vi "Facade 1.vi"(0 "Data In":T7, 2 "Display State In":T4, 3 "Container State":T6) -> (6 "Data Out":T7, 7 "Display State Out":T4, 8 "Action":T3)   [LabVIEW 2012, in "paint Xcontrol.xctl"]
doc: "This VI defines the appearance and behavior of the Paint XControl. The front panel of the Facade VI defines the appearance of the XControl. The block diagram of the Facade VI describes the behavior of the XControl, using an Event Structure to defined respones to various events that can occur on the XControl."
uses:
  paint Xcontrol.xctl
  Data 1.ctl
  <vilib>/_xctls/Container State.ctl
  State 1.ctl
  controls/tool enum.ctl
  <vilib>/_xctls/Action.ctl
  <vilib>/Utility/cursorutil.llb/Set Cursor (Icon Pict).vi
  Instance           4 16Saved   Facade 1 .vi
  <vilib>/_xctls/XControlSupport.lvlib
panel:
  in  "Fill Shapes":bool
  in  "Line Style":T1={"Width"=1, "Style"=enum."Solid"}
  in  "Text String":string
  in  "Tool":T2(radio)
  in  "Color":u32(colorbox)
  out "Picture":picture
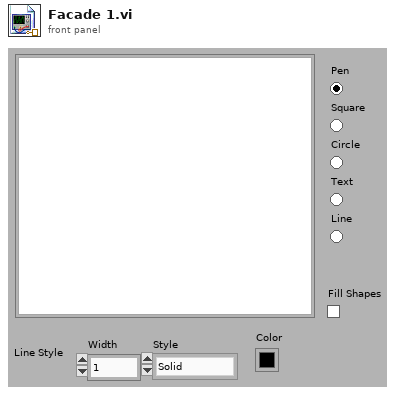
[diagram p1: front panel]
types:
  T1 = cluster{"Width":u16, "Style":enum32{"Solid", "Dash", "Dot", "DashDot", "DashDotDot"}}
  T2 = enum32{"Pen", "Square", "Circle", "Text", "Line"}
  T3 = typedef "XControlSupport.lvlib/Action.ctl" = cluster{"Data Changed?":bool, "State Changed?":bool, "Action Name":string}
  T4 = typedef "paint Xcontrol.xctl/State 1.ctl" = cluster{"Mouse Down?":bool, "Tool":T5, "Start Coords":cluster{"Horizontal":i32, "Vertical":i32}}
  T5 = typedef "paint Xcontrol.xctl/tool enum.ctl" = enum16{"Pen", "Square", "Circle", "Text", "Line"}
  T6 = typedef "XControlSupport.lvlib/Container State.ctl" = cluster{"Indicator?":bool, "Run Mode?":bool, " Refnum":refnum<vi>}
  T7 = typedef "paint Xcontrol.xctl/Data 1.ctl" = picture
  T8 = cluster{"left":i16, "top":i16, "right":i16, "bottom":i16}
  T9 = typedef "LVMouseTypeDef.ctl" = cluster{"Mouse Position":cluster{"X":i32, "Y":i32}, "Mouse Modifiers":cluster{"Button Down":bool, "Shift Mod":bool, "Menu Mod":bool, "Option Mod":bool}}
  T10 = typedef "LVPoint32TypeDef.ctl" = cluster{"Horizontal":i32, "Vertical":i32}
  T11 = typedef "LVPositionTypeDef.ctl" = cluster{"Left":i32, "Top":i32}
  T12 = typedef "LVBoundsTypeDef.ctl" = cluster{"Width":u32, "Height":u32}
  T13 = typedef "imagedata.ctl" = cluster{"image type":i32, "image depth":i32, "image":u8[], "mask":u8[], "colors":u32[], "Rectangle":cluster{"left":i16, "top":i16, "right":i16, "bottom":i16}}
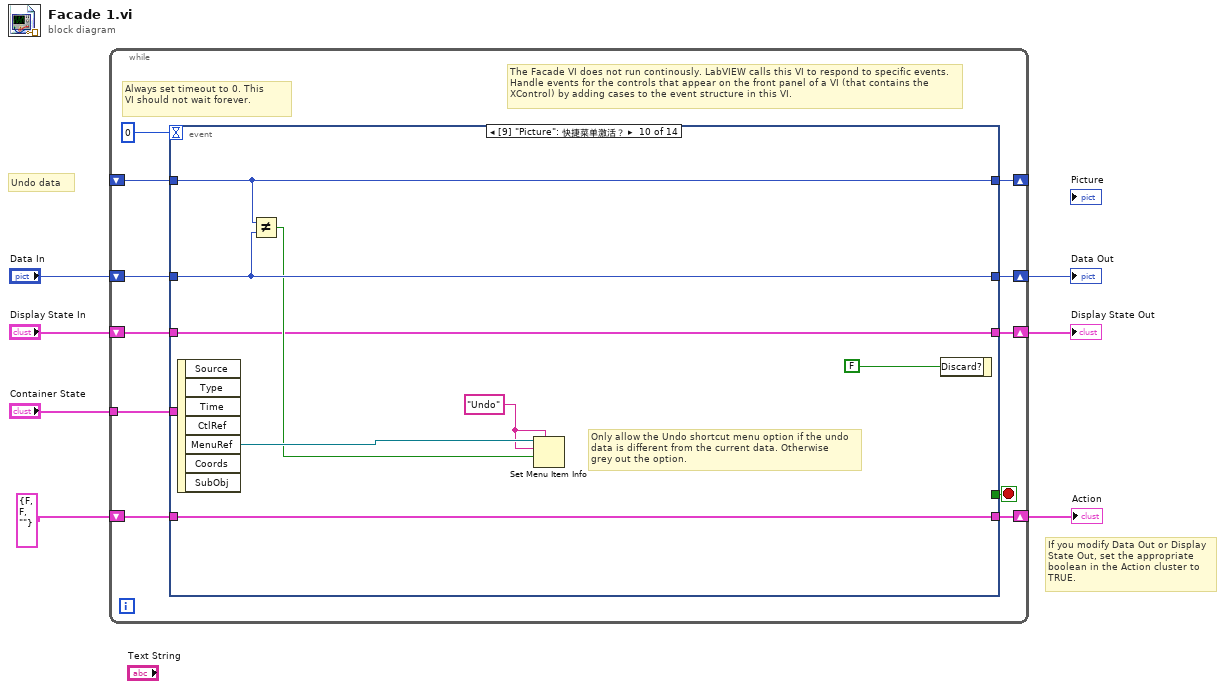
[diagram p0: block diagram]
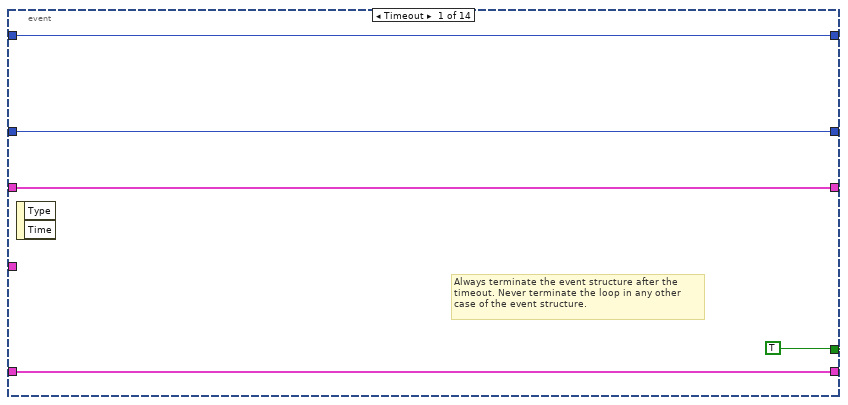
[diagram p2: hidden frame]
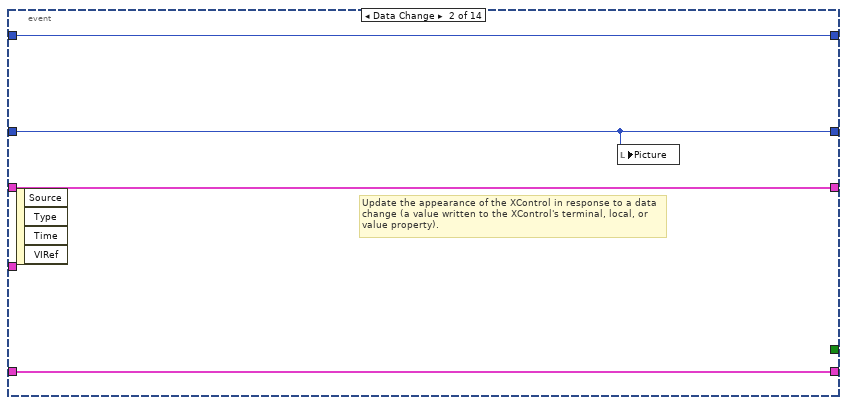
[diagram p3: hidden frame]
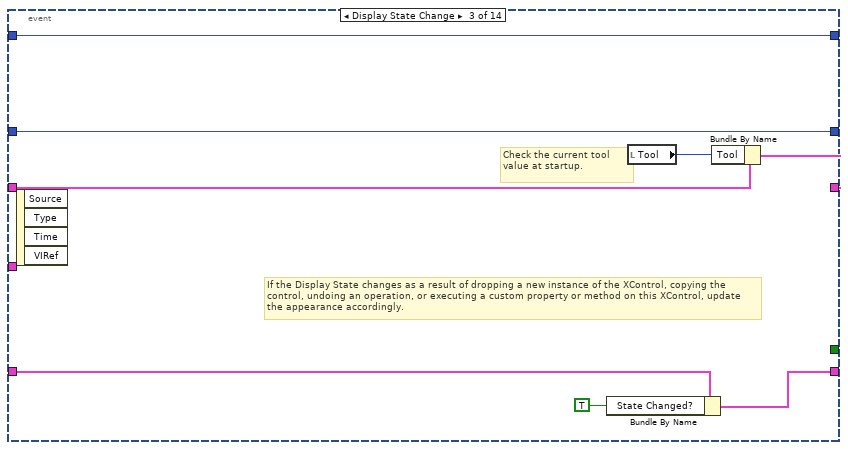
[diagram p4: hidden frame]
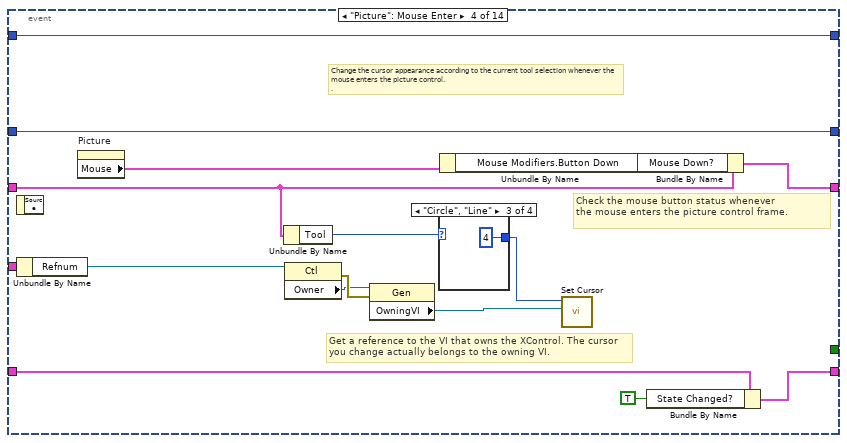
[diagram p5: hidden frame]
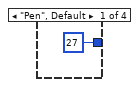
[diagram p6: hidden frame]
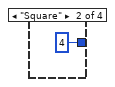
[diagram p7: hidden frame]
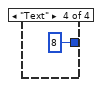
[diagram p8: hidden frame]
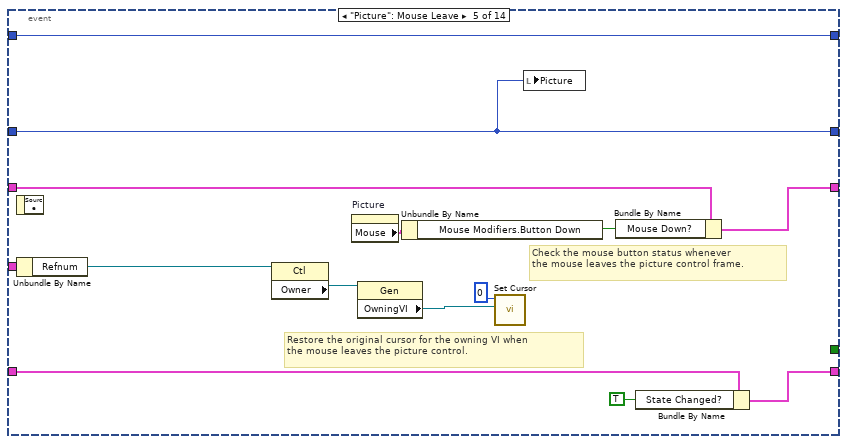
[diagram p9: hidden frame]
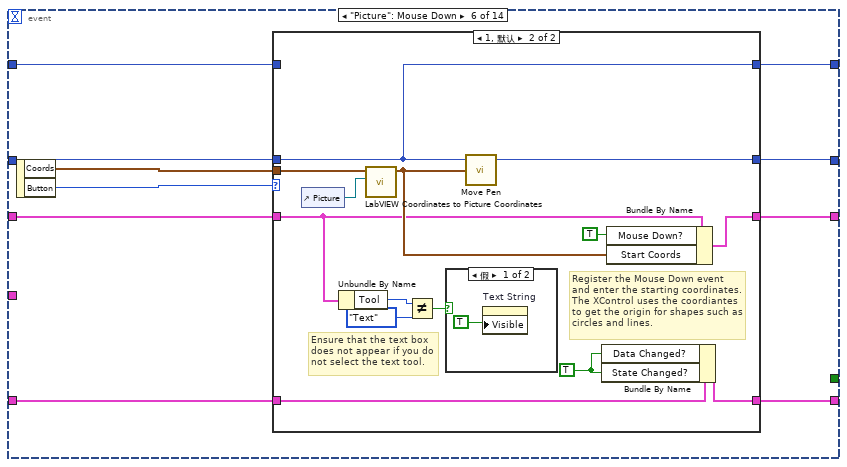
[diagram p10: hidden frame]
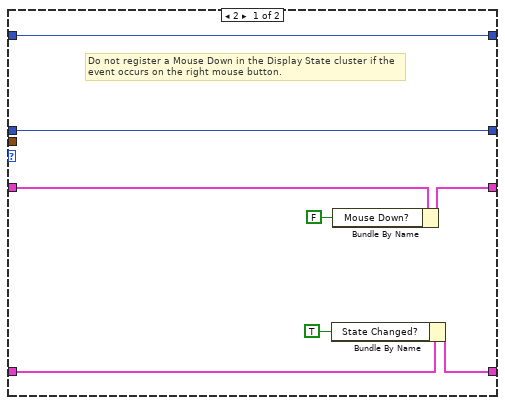
[diagram p11: hidden frame]
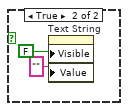
[diagram p12: hidden frame]
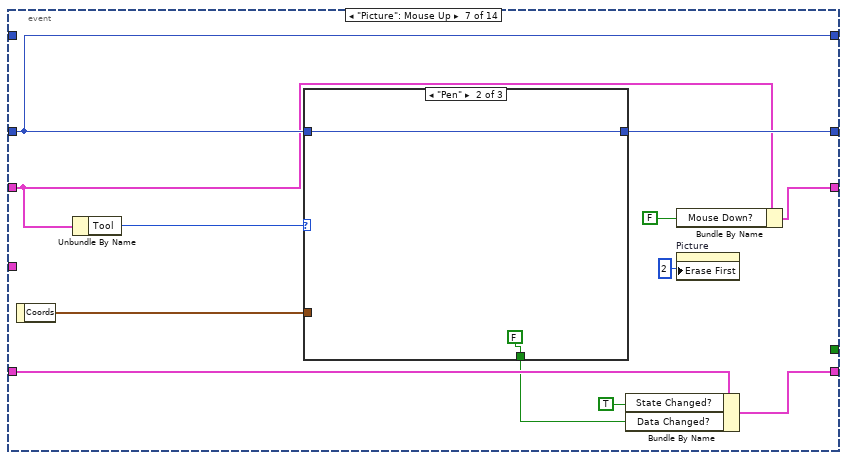
[diagram p13: hidden frame]
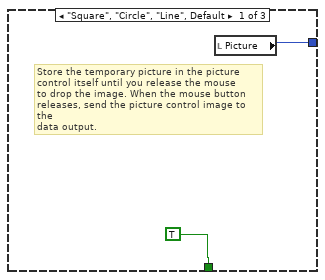
[diagram p14: hidden frame]
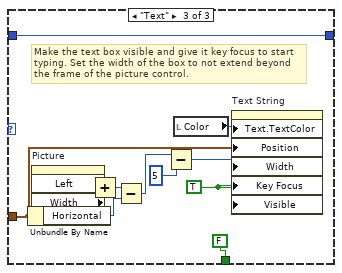
[diagram p15: hidden frame]
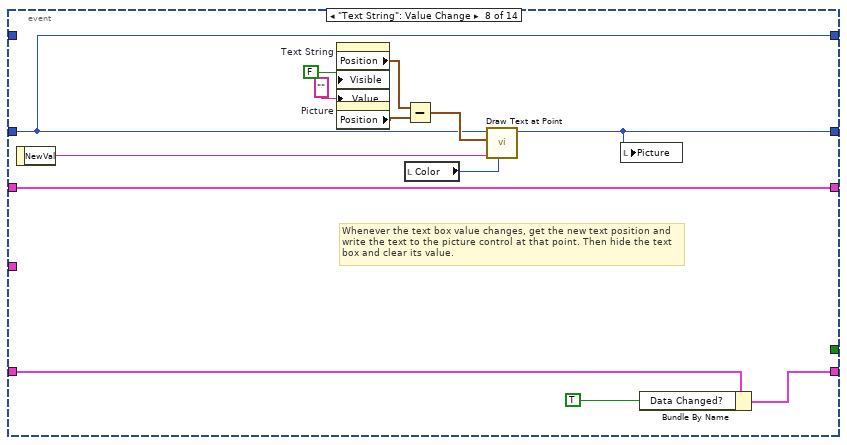
[diagram p16: hidden frame]
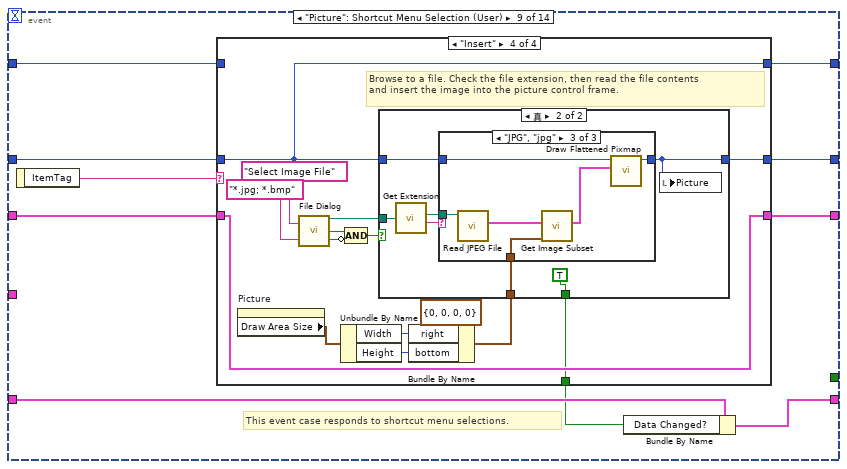
[diagram p17: hidden frame]
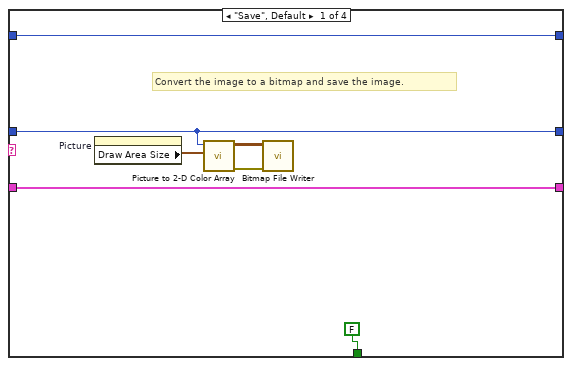
[diagram p18: hidden frame]
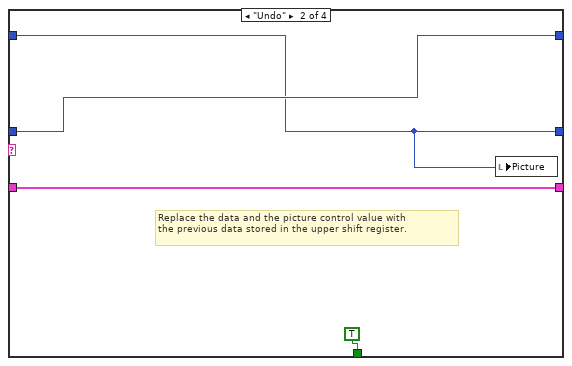
[diagram p19: hidden frame]
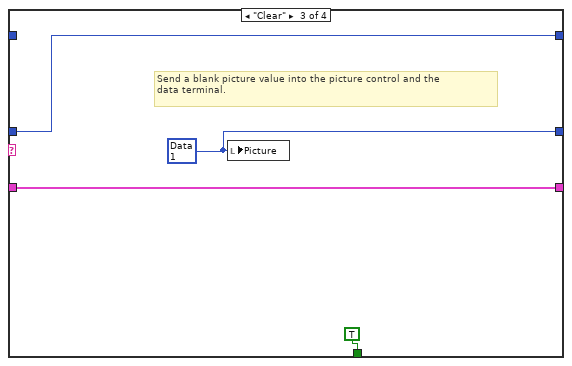
[diagram p20: hidden frame]
diagram:
  # "Undo data"
  # "If you modify Data Out or Display State Out, set the appropriate boolean in the Action cluster to TRUE."
  n1 = while {
    shift-right: [w17] -> w4
    shift-left: "Display State In" -> [w18]
    tunnel: "Container State" -> [w14]
    shift-right: [w13] -> w7
    shift-left: "Data In" -> [w10]
    shift-right: [w11] -> w2
    shift-left: T3 {"Data Changed?"=FALSE, "State Changed?"=FALSE, "Action Name"=""} ("Action") -> [w12]
    shift-right: [w8] -> _
    shift-left: _ -> [w9]
    stop <- w16 stop-if-true
    # "The Facade VI does not run continously. LabVIEW calls this VI to respond to specific events.  Handle events for the controls that appear on the front panel of a VI (that contains the XControl) by adding cases to the event structure in this VI."
    # "Always set timeout to 0. This\nVI should not wait forever."
    n2 = event shown="[9] \"Picture\": 快捷菜单激活？" {
      selector: _ -> [_ _ _ _ _ _ _ _ _ _ _ _ _ _]
      dyn-events: _ -> [_ _ _ _ _ _ _ _ _ _ _ _ _ _]
      timeout: 0 -> [_ _ _ _ _ _ _ _ _ _ _ _ _ _]
      tunnel: w18 -> [w21 w27 w35 w41 w69 w75 w105 w137 w149 w206 w221 w313 w318 w327]
      tunnel: [w21 w27 w34 w47 w68 w76 w115 w137 w148 w206 w221 w313 w318 w326] -> w17
      tunnel: [TRUE _ _ _ _ _ _ _ _ _ _ _ _ _] -> w16
      tunnel: w14 -> [_ _ _ w46 w65 _ _ _ _ _ _ w314 w319 _]
      tunnel: w10 -> [w20 w25 w28 w51 w56 w72 w106 w135 w154 w210 w216 w312 w317 w328]
      tunnel: [w20 w25 w28 w51 w56 w79 w107 w136 w153 w210 w222 w312 w317 w328] -> w13
      tunnel: [w22 w26 w31 w48 w66 w77 w112 w143 w151 w208 w223 w311 w316 w323] -> w11
      tunnel: w12 -> [w22 w26 w32 w50 w67 w78 w114 w145 w152 w208 w224 w311 w316 w325]
      tunnel: w9 -> [w19 w24 w29 w38 w60 w71 _ _ w147 w211 w215 w310 w315 w320]
      tunnel: [w19 w24 w29 w38 w60 w70 w106 w135 w146 w211 w214 w310 w315 w320] -> w8
      event Timeout {
        # "Always terminate the event structure after the timeout. Never terminate the loop in any other case of the event structure."
        n3 = event-data() -> ()  [unwired: 1 in, 2 out]
      }
      event Data Change {
        # "Update the appearance of the XControl in response to a data change (a value written to the XControl's terminal, local, or value property)."
        n4 = event-data() -> ()  [unwired: 1 in, 4 out]
        n5 = local write "Picture"(w25) -> ()
      }
      event Display State Change {
        # "Check the current tool\nvalue at startup."
        # "If the Display State changes as a result of dropping a new instance of the XControl, copying the control, undoing an operation, or executing a custom property or method on this XControl, update the appearance accordingly."
        n6 = event-data() -> ()  [unwired: 1 in, 4 out]
        n7 = Bundle By Name(cluster=w32, "State Changed?"=TRUE) -> (w31:T3)
        n8 = local read "Tool"() -> (w33:T2)
        n9 = Bundle By Name(cluster=w35, "Tool"=w33) -> (w34:T4)
      }
      event "Picture": Mouse Enter {
        # "Check the mouse button status whenever\nthe mouse enters the picture control frame."
        # "Get a reference to the VI that owns the XControl. The cursor you change actually belongs to the owning VI."
        # "Change the cursor appearance according to the current tool selection whenever the mouse enters the picture control.\n."
        n10 = event-data() -> ()  [unwired: 1 in, 1 out]
        n11 = Unbundle By Name(w46) -> ("Refnum"=w45:refnum<vi>)
        n12 = property on="Picture" class="Pict"() -> ("Mouse"=w37:T9)  [unwired: 2 in, 2 out]
        n13 = Unbundle By Name(w41) -> ("Tool"=w40:T5)
        n14 = property class="Ctl"(reference=w45) -> (error out=w44:errorcluster, "Owner"=w43:refnum<vi>)  [unwired: 1 in, 1 out]
        n15 = property class="Gen"(reference=w43, error in=w44) -> ("OwningVI"=w42:refnum<vi>)  [unwired: 2 out]
        n16 = case shown="\"Circle\", \"Line\"" w40 {
          tunnel: [u16 27 ("icon") u16 4 ("icon") u16 4 ("icon") u16 8 ("icon")] -> w39
          frame "Pen", Default {
          }
          frame "Square" {
          }
          frame "Circle", "Line" {
          }
          frame "Text" {
          }
        }
        n17 = Unbundle By Name(w37) -> ("Mouse Modifiers.Button Down"=w36:bool)
        n18 = call-poly <vilib>:"Set Cursor.vi"("VI reference (current VI)"=w42, "icon"=w39) -> ()  [unwired: 8 in, 2 out]
        n19 = Bundle By Name(cluster=w41, "Mouse Down?"=w36) -> (w47:T4)
        n20 = Bundle By Name(cluster=w50, "State Changed?"=TRUE ("Data Changed?")) -> (w48:T3)
      }
      event "Picture": Mouse Leave {
        # "Check the mouse button status whenever\nthe mouse leaves the picture control frame."
        # "Restore the original cursor for the owning VI when\nthe mouse leaves the picture control."
        n21 = event-data() -> ()  [unwired: 1 in, 1 out]
        n22 = Unbundle By Name(w65) -> ("Refnum"=w64:refnum<vi>)
        n23 = property class="Ctl"(reference=w64) -> ("Owner"=w63:refnum<vi>)  [unwired: 1 in, 2 out]
        n24 = property on="Picture" class="Pict"() -> ("Mouse"=w58:T9)  [unwired: 2 in, 2 out]
        n25 = property class="Gen"(reference=w63) -> ("OwningVI"=w62:refnum<vi>)  [unwired: 1 in, 2 out]
        n26 = Unbundle By Name(w58) -> ("Mouse Modifiers.Button Down"=w57:bool)
        n27 = call-poly <vilib>:"Set Cursor.vi"("VI reference (current VI)"=w62, "icon"=u16 0) -> ()  [unwired: 8 in, 2 out]
        n28 = local write "Picture"(w56) -> ()
        n29 = Bundle By Name(cluster=w69, "Mouse Down?"=w57) -> (w68:T4)
        n30 = Bundle By Name(cluster=w67, "State Changed?"=TRUE ("Data Changed?")) -> (w66:T3)
      }
      event "Picture": Mouse Down {
        n31 = event-data() -> ("Coords"=w74:T10, "Button"=w73:u16)  [unwired: 1 in]
        n32 = case shown="1, 默认" w73 {
          tunnel: w72 -> [w87 w88]
          tunnel: [w87 w89] -> w79
          tunnel: w78 -> [w84 w100]
          tunnel: [w82 w99] -> w77
          tunnel: [w81 w97] -> w76
          tunnel: w75 -> [w86 w94]
          tunnel: w74 -> [_ w95]
          tunnel: w71 -> [w80 _]
          tunnel: [w80 w88] -> w70
          frame 2 {
            # "Do not register a Mouse Down in the Display State cluster if the event occurs on the right mouse button."
            n33 = Bundle By Name(cluster=w84, "State Changed?"=TRUE) -> (w82:T3)
            n34 = Bundle By Name(cluster=w86, "Mouse Down?"=FALSE) -> (w81:T4)
          }
          frame 1, Default {
            w90 = TRUE ("Data Changed?")
            # "Ensure that the text box does not appear if you do not select the text tool."
            # "Register the Mouse Down event and enter the starting coordinates. The XControl uses the coordiantes to get the origin for shapes such as circles and lines."
            n35 = control-ref of="Picture"() -> (w101:refnum<vi>)
            n36 = Unbundle By Name(w94) -> ("Tool"=w93:T5)
            n37 = call "LabVIEW Coordinates to Picture Coordinates.vi"("CtlRef"=w101, "LabVIEW Coordinates"=w95) -> ("Picture Control Coordinates"=w96:cluster{"Horizontal":i32, "Vertical":i32})  [unwired: 8 in, 1 out]
            n38 = Not Equal?(x=w93, y=tool_enum."Text") -> (x != y?=w91:bool)
            n39 = case shown="假" w91 {
              frame False {
                n40 = property on="Text String" class="Str"("Visible"=TRUE) -> ()  [unwired: 2 in, 2 out]
              }
              frame True {
                n41 = property on="Text String" class="Str"("Visible"=FALSE, "Value"="" ("Text String")) -> ()  [unwired: 2 in, 2 out]
              }
            }
            n42 = call <vilib>:"Move Pen.vi"("new position"=w96, "picture"=w88) -> ("new picture"=w89:picture)  [unwired: 3 in]
            n43 = Bundle By Name(cluster=w100, "Data Changed?"=w90, "State Changed?"=w90) -> (w99:T3)
            n44 = Bundle By Name(cluster=w94, "Mouse Down?"=TRUE, "Start Coords"=w96) -> (w97:T4)
          }
        }
      }
      event "Picture": Mouse Up {
        n45 = event-data() -> ("Coords"=w108:T10)  [unwired: 1 in]
        n46 = Unbundle By Name(w105) -> ("Tool"=w111:T5)
        n47 = case shown="\"Pen\"" w111 {
          tunnel: w106 -> [_ w120 w132]
          tunnel: [w118 w120 w132] -> w107
          tunnel: [TRUE ("State Changed?") FALSE ("State Changed?") FALSE ("State Changed?")] -> w110
          tunnel: w108 -> [_ _ w128]
          frame "Square", "Circle", "Line", Default {
            # "Store the temporary picture in the picture control itself until you release the mouse\nto drop the image. When the mouse button\nreleases, send the picture control image to the\ndata output."
            n48 = local read "Picture"() -> (w118:picture)
          }
          frame "Pen" {
          }
          frame "Text" {
            w130 = TRUE ("Key Focus")
            # "Make the text box visible and give it key focus to start typing. Set the width of the box to not extend beyond the frame of the picture control."
            n49 = Unbundle By Name(w128) -> ("Horizontal"=w124:i32)
            n50 = property on="Picture" class="Pict"() -> ("Left"=w127:i32, "Width"=w126:u32)  [unwired: 2 in, 2 out]
            n51 = Add(x=w127, y=w126) -> (x+y=w125:u32)
            n52 = Subtract(x=w125, y=w124) -> (x-y=w123:u32)
            n53 = Subtract(x=w123, y=u32 5) -> (x-y=w121:u32)
            n54 = local read "Color"() -> (w129:u32)
            n55 = property on="Text String" class="Str"("Text.TextColor"=w129, "Position"=w128, "Width"=w121, "Key Focus"=w130, "Visible"=w130) -> ()  [unwired: 2 in, 2 out]
          }
        }
        n56 = Bundle By Name(cluster=w114, "State Changed?"=TRUE, "Data Changed?"=w110) -> (w112:T3)
        n57 = Bundle By Name(cluster=w105, "Mouse Down?"=FALSE) -> (w115:T4)
        n58 = property on="Picture" class="Pict"("Erase First"=u8 2) -> ()  [unwired: 2 in, 2 out]
      }
      event "Text String": Value Change {
        # "Whenever the text box value changes, get the new text position and write the text to the picture control at that point. Then hide the text box and clear its value."
        n59 = event-data() -> ("NewVal"=w142:string)  [unwired: 1 in]
        n60 = property on="Text String" class="Str"("Visible"=FALSE, "Value"="" ("Text String")) -> ("Position"=w141:T11)  [unwired: 2 in, 2 out]
        n61 = property on="Picture" class="Pict"() -> ("Position"=w140:T11)  [unwired: 2 in, 2 out]
        n62 = Subtract(x=w141, y=w140) -> (x-y=w139:T11)
        n63 = local read "Color"() -> (w138:u32)
        n64 = call <vilib>:"Draw Text at Point.vi"("text color(black)"=w138, "text"=w142, "origin"=w139, "picture"=w135) -> ("new picture"=w136:picture)  [unwired: 6 in, 1 out]
        n65 = local write "Picture"(w136) -> ()
        n66 = Bundle By Name(cluster=w145, "Data Changed?"=TRUE) -> (w143:T3)
      }
      event "Picture": Shortcut Menu Selection (User) {
        # "This event case responds to shortcut menu selections."
        n67 = event-data() -> ("ItemTag"=w155:string)  [unwired: 1 in]
        n68 = case shown="\"Insert\"" w155 {
          tunnel: w154 -> [w159 w164 w167 w176]
          tunnel: [w159 w163 w170 w179] -> w153
          tunnel: [FALSE TRUE TRUE w177] -> w150
          tunnel: w149 -> [w157 w166 w168 w178]
          tunnel: [w157 w166 w168 w178] -> w148
          tunnel: w147 -> [w156 w163 _ _]
          tunnel: [w156 w164 w167 w176] -> w146
          frame "Save", Default {
            # "Convert the image to a bitmap and save the image."
            n69 = property on="Picture" class="Pict"() -> ("Draw Area Size"=w162:T12)  [unwired: 2 in, 2 out]
            n70 = call "Picture to 2-D Color Array.vi"("input cluster"=w162, "picture"=w159) -> ("error out"=w160:errorcluster, "Color Array"=w161:cluster{"Red":u8, "Green":u8, "Blue":u8}[][])  [unwired: 8 in]
            n71 = call "Bitmap File Writer.vi"("error in"=w160, "Color Array"=w161) -> ()  [unwired: 9 in, 1 out]
          }
          frame "Undo" {
            # "Replace the data and the picture control value with\nthe previous data stored in the upper shift register."
            n72 = local write "Picture"(w163) -> ()
          }
          frame "Clear" {
            w170 = T7 data[5B] ("Data In")
            # "Send a blank picture value into the picture control and the\ndata terminal."
            n73 = local write "Picture"(w170) -> ()
          }
          frame "Insert" {
            # "Browse to a file. Check the file extension, then read the file contents\nand insert the image into the picture control frame."
            n74 = property on="Picture" class="Pict"() -> ("Draw Area Size"=w174:T12)  [unwired: 2 in, 2 out]
            n75 = call "File Dialog"("prompt"="Select Image File", "pattern (all files)"="*.jpg; *.bmp") -> ("selected path"=w180:path, "exists"=w183:bool, "cancelled"=w182:bool)  [unwired: 10 in, 1 out]
            n76 = Unbundle By Name(w174) -> ("Width"=w173:u32, "Height"=w172:u32)
            n77 = Compound Arithmetic op=AND(w183, invert w182) -> (w181:bool)
            n78 = Bundle By Name(cluster=T8 {"left"=0, "top"=0, "right"=0, "bottom"=0} ("rect"), "right"=w173, "bottom"=w172) -> (w171:T8)
            n79 = case shown="真" w181 {
              tunnel: w180 -> [_ w194]
              tunnel: w176 -> [w187 w191]
              tunnel: [w187 w189] -> w179
              tunnel: [FALSE TRUE] -> w177
              tunnel: w171 -> [_ w188]
              frame False {
              }
              frame True {
                n80 = call "Get Extension.vi"("Path In"=w194) -> ("Duplicate Path Out"=w192:path, "Extension"=w193:string)  [unwired: 8 in]
                n81 = case shown="\"JPG\", \"jpg\"" w193 {
                  tunnel: w192 -> [w196 _ w205]
                  tunnel: w191 -> [w198 w199 w204]
                  tunnel: [w197 w199 w203] -> w189
                  tunnel: w188 -> [_ _ w201]
                  frame "BMP", "bmp" {
                    n82 = call <vilib>:"Read BMP File.vi"("path to BMP file"=w196) -> ("image data"=w195:T13)  [unwired: 8 in, 2 out]
                    n83 = call <vilib>:"Draw Flattened Pixmap.vi"("image data"=w195, "picture"=w198) -> ("new picture"=w197:picture)  [unwired: 7 in]
                  }
                  frame Default {
                  }
                  frame "JPG", "jpg" {
                    n84 = call <vilib>:"Read JPEG File.vi"("path to JPEG file"=w205) -> ("image data"=w202:T13)  [unwired: 8 in, 2 out]
                    n85 = call <vilib>:"Get Image Subset.vi"("subset rect"=w201, "image data"=w202) -> ("image subset"=w200:T13)  [unwired: 4 in, 1 out]
                    n86 = call <vilib>:"Draw Flattened Pixmap.vi"("image data"=w200, "picture"=w204) -> ("new picture"=w203:picture)  [unwired: 7 in]
                  }
                }
                n87 = local write "Picture"(w189) -> ()
              }
            }
          }
        }
        n88 = Bundle By Name(cluster=w152, "Data Changed?"=w150) -> (w151:T3)
      }
      event "Picture": Shortcut Menu Activation? {
        w212 = "Undo" ("item name")
        # "Only allow the Undo shortcut menu option if the undo data is different from the current data. Otherwise\ngrey out the option."
        n89 = event-data() -> ("MenuRef"=w213:refnum<k9>)  [unwired: 1 in, 6 out]
        n90 = Not Equal?(x=w211, y=w210) -> (x != y?=w209:bool)
        n91 = Set Menu Item Info(7:w212, 9:w209, 10:w212, 11:w213) -> ()  [unwired: 3 in, 2 out]
        n92 = event-data("Discard?"=FALSE) -> ()  [unwired: 1 in, 1 out]
      }
      event "Picture": Mouse Move {
        n93 = event-data() -> ("Coords"=w227:T10, "CtlRef"=w226:refnum<vi>)  [unwired: 1 in]
        n94 = Unbundle By Name(w221) -> ("Tool"=w220:T5, "Mouse Down?"=w225:bool, "Start Coords"=w219:cluster{"Horizontal":i32, "Vertical":i32})
        n95 = case shown="真" w225 {
          tunnel: [w230 w238] -> w222
          tunnel: w227 -> [_ w242]
          tunnel: w226 -> [_ w243]
          tunnel: w216 -> [w230 w241]
          tunnel: w224 -> [w229 w240]
          tunnel: [w229 w239] -> w223
          tunnel: w220 -> [_ w237]
          tunnel: w219 -> [_ w236]
          tunnel: "Line Style" -> [_ w234]
          tunnel: "Fill Shapes" -> [_ w233]
          tunnel: w215 -> [w228 w232]
          tunnel: [w228 w231] -> w214
          frame False {
            # "Do not take action unless the mouse button is currently down."
          }
          frame True {
            n96 = case shown="\"Square\"" w237 {
              tunnel: w243 -> [w253 w272 w294 _ w306]
              tunnel: w242 -> [w252 w271 w295 _ w307]
              tunnel: w241 -> [w245 w274 w293 w298 w303]
              tunnel: w240 -> [w251 w258 w287 w297 w301]
              tunnel: [w250 w258 w287 w297 w301] -> w239
              tunnel: [w244 w274 w293 w298 w303] -> w238
              tunnel: w236 -> [_ w269 w284 _ w309]
              tunnel: [w244 w257 w292 w298 w302] -> w235
              tunnel: w234 -> [w246 w256 w277 _ w300]
              tunnel: w233 -> [_ w255 w276 _ _]
              tunnel: w232 -> [_ w254 w275 w296 w299]
              tunnel: [w245 w254 w275 w296 w299] -> w231
              frame "Pen", Default {
                # "Draw pen marks at the current location."
                n97 = call "LabVIEW Coordinates to Picture Coordinates.vi"("CtlRef"=w253, "LabVIEW Coordinates"=w252) -> ("Picture Control Coordinates"=w248:cluster{"Horizontal":i32, "Vertical":i32})  [unwired: 8 in, 1 out]
                n98 = call <vilib>:"Draw Line.vi"("picture"=w245, "end point"=w248, "color(black)"="Color", "pen"=w246) -> ("new picture"=w244:picture)  [unwired: 5 in]
                n99 = Bundle By Name(cluster=w251, "Data Changed?"=TRUE) -> (w250:T3)
              }
              frame "Square" {
                # "Draw a square using the start coordinates to determine the origin. Output the new picture to the picture control but not to the data terminal. Only drop the image when the mouse button releases."
                n100 = call "LabVIEW Coordinates to Picture Coordinates.vi"("CtlRef"=w272, "LabVIEW Coordinates"=w271) -> ("Picture Control Coordinates"=w268:cluster{"Horizontal":i32, "Vertical":i32})  [unwired: 8 in, 1 out]
                n101 = Unbundle(w269) -> ("Horizontal"=w267:i32, "Vertical"=w265:i32)
                n102 = Unbundle(w268) -> ("Horizontal"=w266:i32, "Vertical"=w264:i32)
                n103 = Max & Min(x=w265, y=w264) -> (max(x,y)=w261:i32, min(x,y)=w260:i32)
                n104 = Max & Min(x=w267, y=w266) -> (max(x,y)=w263:i32, min(x,y)=w262:i32)
                n105 = local read "Color"() -> (w273:u32)
                n106 = Bundle(cluster=T8 {"left"=0, "top"=0, "right"=0, "bottom"=0} ("rect"), "left"=w262, "top"=w260, "right"=w263, "bottom"=w261) -> (w259:T8)
                n107 = call <vilib>:"Draw Rect.vi"("picture"=w274, "rect"=w259, "fill?(F)"=w255, "color(black)"=w273, "pen"=w256) -> ("new picture"=w257:picture)  [unwired: 4 in]
              }
              frame "Circle" {
                # "Draw a circle using the start coordinates to determine the\norigin. Output the new picture to the picture control but\nnot to the data terminal. Only drop the image when the\nmouse button releases."
                n108 = call "LabVIEW Coordinates to Picture Coordinates.vi"("CtlRef"=w294, "LabVIEW Coordinates"=w295) -> ("Picture Control Coordinates"=w285:cluster{"Horizontal":i32, "Vertical":i32})  [unwired: 8 in, 1 out]
                n109 = Unbundle By Name(w284) -> ("Horizontal"=w291:i32)
                n110 = Unbundle By Name(w285) -> ("Horizontal"=w290:i32)
                n111 = Add(x=w285, y=w284) -> (x+y=w283:cluster{"Horizontal":i32, "Vertical":i32})
                n112 = Max & Min(x=w291, y=w290) -> (max(x,y)=w289:i32, min(x,y)=w288:i32)
                n113 = Quotient & Remainder(x=w283, y=2) -> (floor(x/y)=w281:cluster{"Horizontal":i32, "Vertical":i32})  [unwired: 1 out]
                n114 = Subtract(x=w289, y=w288) -> (x-y=w280:i32)
                n115 = local read "Color"() -> (w286:u32)
                n116 = Quotient & Remainder(x=w280, y=2) -> (floor(x/y)=w278:i32)  [unwired: 1 out]
                n117 = call <vilib>:"Draw Circle by Radius.vi"("pen"=w277, "color(black)"=w286, "fill?(F)"=w276, "pixel center"=w281, "radius"=w278, "picture"=w293) -> ("new picture"=w292:picture)  [unwired: 5 in]
              }
              frame "Text" {
              }
              frame "Line" {
                # "Draw a line using the start coordinates to determine the\norigin. Output the new picture to the picture control but\nnot to the data terminal. Only drop the image when the\nmouse button releases."
                n118 = call <vilib>:"Move Pen.vi"("new position"=w309, "picture"=w303) -> ("new picture"=w308:picture)  [unwired: 3 in]
                n119 = local read "Color"() -> (w304:u32)
                n120 = call "LabVIEW Coordinates to Picture Coordinates.vi"("CtlRef"=w306, "LabVIEW Coordinates"=w307) -> ("Picture Control Coordinates"=w305:cluster{"Horizontal":i32, "Vertical":i32})  [unwired: 8 in, 1 out]
                n121 = call <vilib>:"Draw Line.vi"("picture"=w308, "end point"=w305, "color(black)"=w304, "pen"=w300) -> ("new picture"=w302:picture)  [unwired: 5 in]
              }
            }
            n122 = local write "Picture"(w235) -> ()
          }
        }
      }
      event Direction Change {
        # "If the direction of the XControl changes from a control to an indicator or vice versa, update the appearance accordingly. This example does not distinguish between a control and an indicator."
        n123 = event-data() -> ()  [unwired: 1 in, 4 out]
        n124 = Unbundle By Name(w314) -> ()  [unwired: 1 out]
      }
      event Exec State Change {
        # "The VI that owns the XControl changed from Edit Mode to Run Mode or vice versa. Update the appearance accordingly. This example does not distinguish between Edit Mode and Run Mode. You can draw on the XControl without running the VI."
        # "Handle the Edit Mode & Run Mode\ncases differently."
        n125 = event-data() -> ()  [unwired: 1 in, 4 out]
        n126 = Unbundle By Name(w319) -> ()  [unwired: 1 out]
      }
      event "Tool": Value Change {
        # "Track any tool value changes. \nSet whether the text box appears and whether to erase first depending on the selected tool."
        n127 = event-data() -> ()  [unwired: 1 in, 6 out]
        n128 = case shown="\"Text\"" "Tool" {
          tunnel: [u8 0 ("Erase First") u8 2 ("Erase First") u8 2 ("Erase First") u8 2 ("Erase First")] -> w322
          frame "Pen", Default {
          }
          frame "Square", "Line" {
          }
          frame "Circle" {
          }
          frame "Text" {
            n129 = property on="Text String" class="Str"("Visible"=FALSE, "Value"="" ("Text String")) -> ()  [unwired: 2 in, 2 out]
          }
        }
        n130 = Bundle By Name(cluster=w327, "Tool"="Tool") -> (w326:T4)
        n131 = Bundle By Name(cluster=w325, "State Changed?"=TRUE) -> (w323:T3)
        n132 = property on="Picture" class="Pict"("Erase First"=w322) -> ()  [unwired: 2 in, 2 out]
      }
    }
  }
  "Display State Out" <- w4
  "Data Out" <- w7
  "Action" <- w2
